vi "send accesspoint cmd.vi"(5 "timeoutMilliseconds":u32, 6 "numLinesToRead":u32, 7 "outputBufferLength":u32, 9 "BYTE_ARRAY":string, 10 "cmdToSend":string, 11 "ap_handle":u32) -> (1 "BYTE_ARRAY out":string, 2 "function return":i32, 3 "ap_handle out":u32)   [LabVIEW 2019, in "apdm.lvlib"]
doc: "APDM_EXPORT int apdm_send_accesspoint_cmd(apdm_ap_handle_t ap_handle,\n const char *cmdToSend, char *BYTE_ARRAY, const uint32_t outputBufferLength,\n const uint32_t numLinesToRead, const uint32_t timeoutMilliseconds);"
uses:
  apdm.lvlib
  Lee Lab/CP FES Walking 2018/Code/Working/LabVIEW/apdm.dll
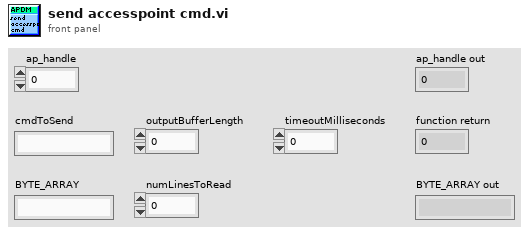
[diagram p1: front panel]
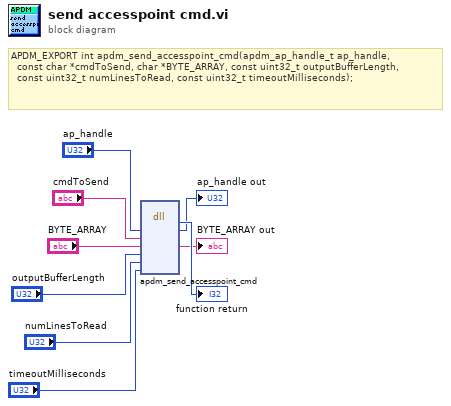
[diagram p0: block diagram]
diagram:
  # "APDM_EXPORT int apdm_send_accesspoint_cmd(apdm_ap_handle_t ap_handle,\n\t\tconst char *cmdToSend, char *BYTE_ARRAY, const uint32_t outputBufferLength,\n\t\tconst uint32_t numLinesToRead, const uint32_t timeoutMilliseconds);"
  n1 = dll-call lib="C:/Users/jfalesi/Dropbox/Lee Lab/CP FES Walking 2018/Code/Working/LabVIEW/apdm.*" fn="apdm_send_accesspoint_cmd"("ap_handle"="ap_handle", "cmdToSend"="cmdToSend", "BYTE_ARRAY"="BYTE_ARRAY", "outputBufferLength"="outputBufferLength", "numLinesToRead"="numLinesToRead", "timeoutMilliseconds"="timeoutMilliseconds") -> (→"function return":i32, "ap_handle"=→"ap_handle out":u32, "BYTE_ARRAY"=→"BYTE_ARRAY out":string)  [unwired: 7 in, 2 out]
